vi "TestInvalidSubpanelRefnum_ErrorOut.vi"(8 "error in (no error)":errorcluster, 11 "TestCase in":refnum<class "TestProtectedSubpanel.lvclass">) -> (0 "error out":errorcluster, 3 "TestCase out":refnum<class "TestProtectedSubpanel.lvclass">)   [LabVIEW 2015, in "TestProtectedSubpanel.lvclass"]
uses:
  TestProtectedSubpanel.lvclass
  TestProtectedSubpanel.lvclass/TestProtectedSubpanel.ctl
  IViewable/IViewable.lvclass/IViewable.ctl
  ProtectedSubpanel/ProtectedSubpanel.lvclass/ProtectedSubpanel.ctl
  ProtectedSubpanel/Evaluate Insertion Request.vi
  IViewable/Evaluate Destination Subpanel.vi
  ProtectedSubpanel/Do Insertion.vi
  IViewable/IViewable.lvclass
  ProtectedSubpanel/ProtectedSubpanel.lvclass
panel:
  out "Insert Error":errorcluster
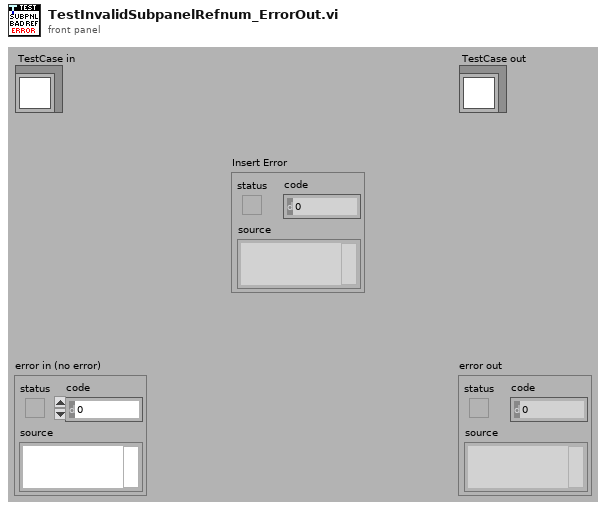
[diagram p1: front panel]
types:
  T1 = typedef "IViewable.lvlib/ProtectedSubpanel.lvclass/Protected Subpanel Reference.ctl" = refnum<data-value>
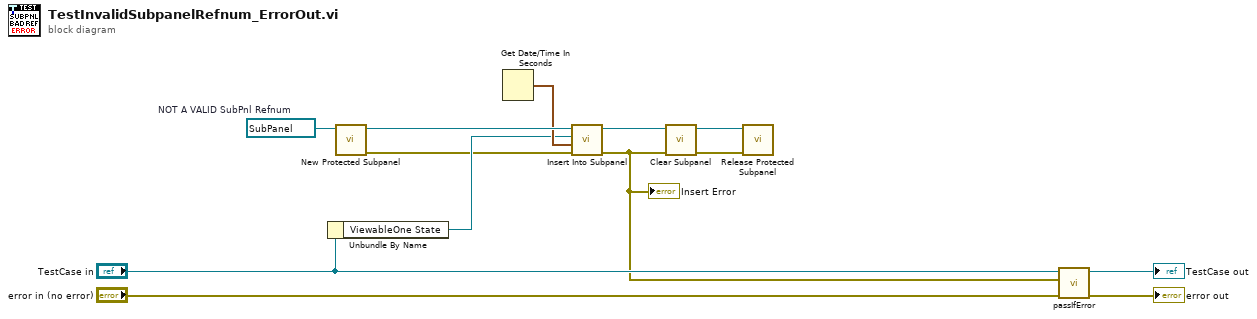
[diagram p0: block diagram]
diagram:
  w1 = refnum<vi> refnum  # NOT A VALID SubPnl Refnum
  n1 = Unbundle By Name("TestCase in") -> ("ViewableOne State"=w7:refnum<class "IViewable.lvclass">)
  n2 = call "New Protected Subpanel.vi"("SubPnl Refnum"=w1) -> ("error out"=w6:errorcluster, "Protected Subpanel"=w10:T1)  [unwired: 9 in]
  n3 = Get Date/Time In Seconds() -> (seconds since 1Jan1904=w9:timestamp)
  n4 = call "Insert Into Subpanel.vi"("error in (no error)"=w6, "Insertion Request Time"=w9, "Viewable"=w7, "Protected Subpanel"=w10) -> ("error out"=w5:errorcluster, "Protected Subpanel"=w4:T1)  [unwired: 4 in, 2 out]
  "Insert Error" <- w5
  n5 = call "Clear Subpanel.vi"("error in (no error)"=w5, "Protected Subpanel"=w4) -> ("error out"=w2:errorcluster, "Protected Subpanel Out"=w3:T1)  [unwired: 8 in]
  n6 = call "Release Protected Subpanel.vi"("error in (no error)"=w2, "Protected Subpanel"=w3) -> ()  [unwired: 9 in, 1 out]
  n7 = call-dynamic "passIfError.vi"("error in (no error)"="error in (no error)", "error"=w5, "TestCase in"="TestCase in") -> ("error out"=→"error out":errorcluster, "TestCase out"=→"TestCase out":refnum<class "TestProtectedSubpanel.lvclass">)  [unwired: 7 in]
